vi "FGV_FPGA_ref_4ch.vi"(7 "Action":T2(ring), 8 "error in (no error)":errorcluster) -> (0 "error out":errorcluster, 3 "FPGA VI Reference Out":T1)   [LabVIEW 2020]
uses:
  FPGA_ref.ctl
  Globals/FPGA Globals.vi
  <vilib>/FPGAPlugInAG/PXIe-7976R/niLvFpga_Open_PXIe-7976R.vi
  <vilib>/rvi/interface/common/dynamic/niFpgaDynamicAddResources.vi
  <vilib>/FPGAPlugInAG/PXIe-7975R/niLvFpga_Open_PXIe-7975R.vi
  <vilib>/FPGAPlugInAG/PXIe-7966R/niLvFpga_Open_PXIe-7966R.vi
  <vilib>/FPGAPlugInAG/Dynamic/niLvFpga_Close_Dynamic.vi
  <vilib>/rvi/interface/nirviOpenFPGA/nirviOpenFPGA.xnode
  FPGA Bitfiles/aolcontrolprojec_FPGATarget_ContTrigpuls_7976_5772DC.lvbitx
  FPGA Bitfiles/aolcontrolprojec_FPGATarget_ContTrigpuls_7976_5772AC.lvbitx
  FPGA Bitfiles/aolcontrolprojec_FPGATarget_ContTrigpuls_7975_5772AC.lvbitx
  FPGA Bitfiles/aolcontrolprojec_FPGATarget_ContTrigpuls_7966_5772DC.lvbitx
  FPGA Bitfiles/aolcontrolprojec_FPGATarget_ContTrigpuls_7966_5772AC.lvbitx
  <vilib>/rvi/interface/nirviCloseFPGA/nirviCloseFPGA.xnode
  FPGA Bitfiles/aolcontrolprojec_FPGATarget_GenerateTrigpuls_kZV7cFEd9rk.lvbitx
panel:
  in  "Local":bool
  in  "FPGA Card":enum16{"7976R", "7975R"}(ring)
  in  "Adapter Module":enum16{"5772-DC", "5772-AC"}(ring)
  in  "RIO Resource Name":string
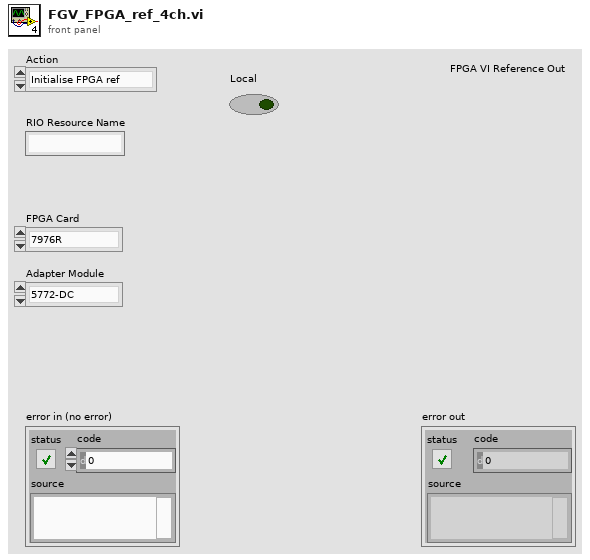
[diagram p1: front panel]
types:
  T1 = typedef "FPGA_ref.ctl" = refnum<k20>
  T2 = enum16{"Initialise FPGA ref", "Read FPGA ref", "Close FPGA Ref"}
  T3 = typedef "FPGA_DAQ_settings.ctl" = cluster{"Use FlexRIO Trigger":bool, "RIO Resource Name":string, "Use detected RIO resource":bool, "Ethernet Card WinPCap Port ":i16, "Adapter Module":T4, "FPGA Card":T5}
  T4 = typedef "FPGA_adapter_type.ctl" = enum16{"5772-DC", "5772-AC"}
  T5 = typedef "FPGA_card_type.ctl" = enum16{"7976R", "7975R", "7966R"}
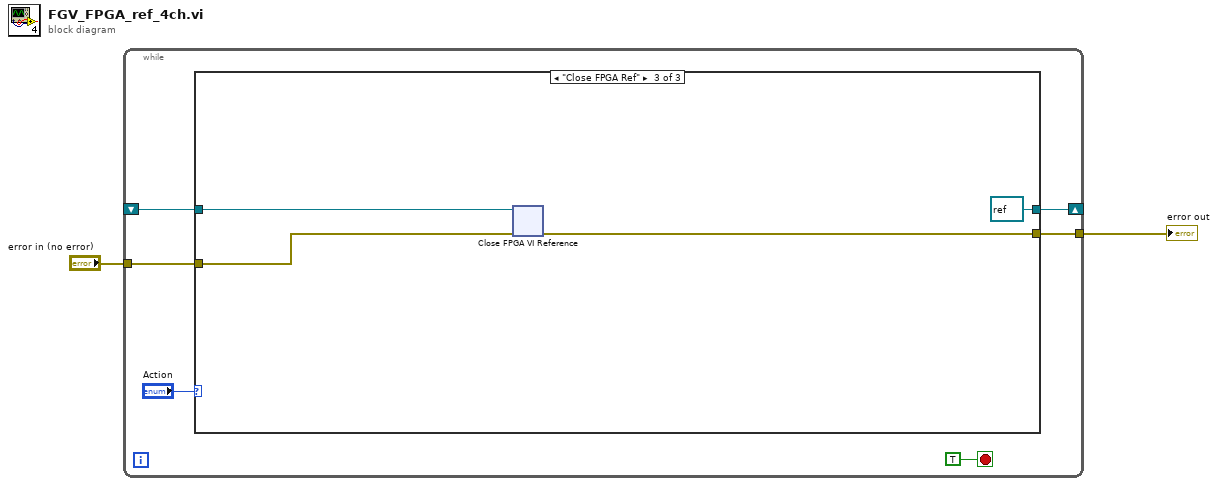
[diagram p0: block diagram]
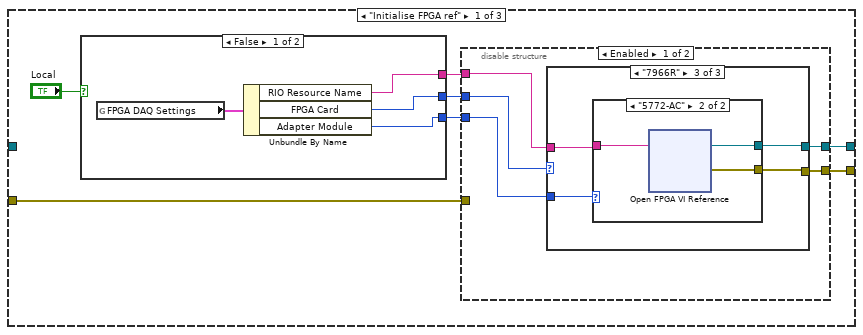
[diagram p2: hidden frame]
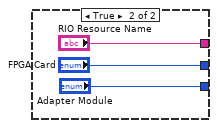
[diagram p3: hidden frame]
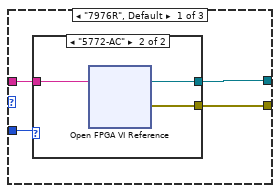
[diagram p4: hidden frame]
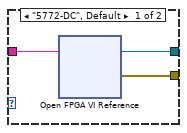
[diagram p5: hidden frame]
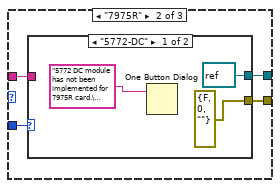
[diagram p6: hidden frame]
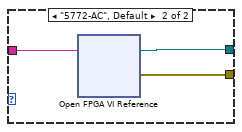
[diagram p7: hidden frame]
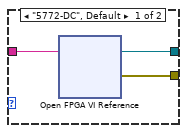
[diagram p8: hidden frame]
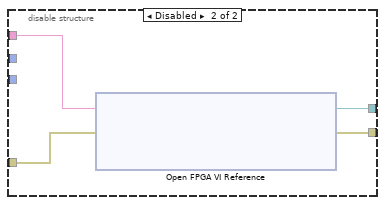
[diagram p9: hidden frame]
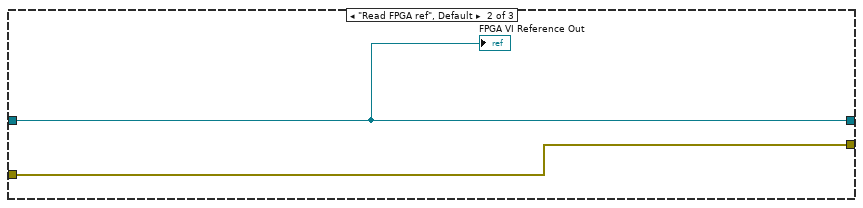
[diagram p10: hidden frame]
diagram:
  n1 = while {
    shift-right: [w6] -> _
    shift-left: _ -> [w5]
    tunnel: [w4] -> w1
    tunnel: "error in (no error)" -> [w3]
    stop <- TRUE stop-if-true
    n2 = case shown="\"Close FPGA Ref\"" "Action" {
      tunnel: [w12 w63 refnum<k20> refnum ("FPGA VI Reference Out")] -> w6
      tunnel: w5 -> [_ w63 w67]
      tunnel: [w11 w62 w65] -> w4
      tunnel: w3 -> [w10 w62 w66]
      frame "Initialise FPGA ref" {
        n3 = case shown="False" "Local" {
          tunnel: [w18 "RIO Resource Name"] -> w15
          tunnel: [w16 "Adapter Module"] -> w14
          tunnel: [w17 "FPGA Card"] -> w13
          frame False {
            n4 = global read "FPGA Globals.vi" "FPGA DAQ Settings"() -> (w19:T3)
            n5 = Unbundle By Name(w19) -> ("RIO Resource Name"=w18:string, "FPGA Card"=w17:T5, "Adapter Module"=w16:T4)
          }
          frame True {
          }
        }
        n6 = disable-structure shown="Enabled" {
          disable-tunnel: w15 -> [w27 w59]
          disable-tunnel: w14 -> [w26 _]
          disable-tunnel: w13 -> [w25 _]
          disable-tunnel: [w24 w60] -> w11
          disable-tunnel: [w23 w61] -> w12
          disable-tunnel: w10 -> [_ w58]
          frame Enabled {
            n7 = case shown="\"7966R\"" w25 {
              tunnel: [w31 w40 w49] -> w23
              tunnel: [w30 w39 w48] -> w24
              tunnel: w26 -> [w29 w41 w51]
              tunnel: w27 -> [w28 w38 w50]
              frame "7976R", Default {
                n8 = case shown="\"5772-AC\"" w29 {
                  tunnel: [w34 w37] -> w31
                  tunnel: [w33 w36] -> w30
                  tunnel: w28 -> [w32 w35]
                  frame "5772-DC", Default {
                    n9 = xnode "Open FPGA VI Reference"("resource name"=w32) -> ("FPGA VI Reference Out"=w34:refnum<k20>, "error out"=w33:errorcluster)  [unwired: 1 in]
                  }
                  frame "5772-AC" {
                    n10 = xnode "Open FPGA VI Reference"("resource name"=w35) -> ("FPGA VI Reference Out"=w37:refnum<k20>, "error out"=w36:errorcluster)  [unwired: 1 in]
                  }
                }
              }
              frame "7975R" {
                n11 = case shown="\"5772-DC\"" w41 {
                  tunnel: [refnum<k20> refnum ("FPGA VI Reference Out") w47] -> w40
                  tunnel: [errorcluster {"status"=FALSE, "code"=0, "source"=""} ("error out") w46] -> w39
                  tunnel: w38 -> [_ w45]
                  frame "5772-DC" {
                    n12 = One Button Dialog(message="5772 DC module has not been implemented for 7975R card.\nPlease check your installed hardware. ") -> ()  [unwired: 1 in, 1 out]
                  }
                  frame "5772-AC", Default {
                    n13 = xnode "Open FPGA VI Reference"("resource name"=w45) -> ("FPGA VI Reference Out"=w47:refnum<k20>, "error out"=w46:errorcluster)  [unwired: 1 in]
                  }
                }
              }
              frame "7966R" {
                n14 = case shown="\"5772-AC\"" w51 {
                  tunnel: [w54 w57] -> w49
                  tunnel: [w53 w56] -> w48
                  tunnel: w50 -> [w52 w55]
                  frame "5772-DC", Default {
                    n15 = xnode "Open FPGA VI Reference"("resource name"=w52) -> ("FPGA VI Reference Out"=w54:refnum<k20>, "error out"=w53:errorcluster)  [unwired: 1 in]
                  }
                  frame "5772-AC" {
                    n16 = xnode "Open FPGA VI Reference"("resource name"=w55) -> ("FPGA VI Reference Out"=w57:refnum<k20>, "error out"=w56:errorcluster)  [unwired: 1 in]
                  }
                }
              }
            }
          }
          frame Disabled {
            n17 = xnode "Open FPGA VI Reference"("error in"=w58, "resource name"=w59) -> ("FPGA VI Reference Out"=w61:refnum<k20>, "error out"=w60:errorcluster)
          }
        }
      }
      frame "Read FPGA ref", Default {
        "FPGA VI Reference Out" <- w63
      }
      frame "Close FPGA Ref" {
        n18 = xnode "Close FPGA VI Reference"("FPGA VI Reference In"=w67, "error in"=w66) -> ("error out"=w65:errorcluster)
      }
    }
  }
  "error out" <- w1
